vi "IHM_GetStringValue.vi"(4 "error in (no error)":errorcluster caption="entrée d'erreur (pas d'erreur)", 7 "Ref_IN":T1) -> (0 "Error out":errorcluster, 2 "StringValue":string, 3 "Ref_OUT":T1)   [LabVIEW 2013]
panel:
  out "ClassName":string
  out "Name":string
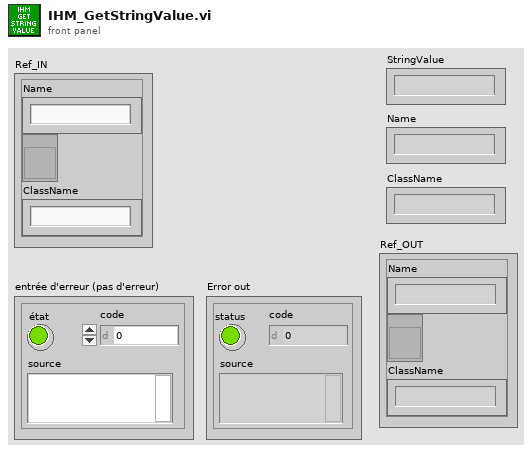
[diagram p1: front panel]
types:
  T1 = cluster{"Name":string, refnum<vi>, "ClassName":string}
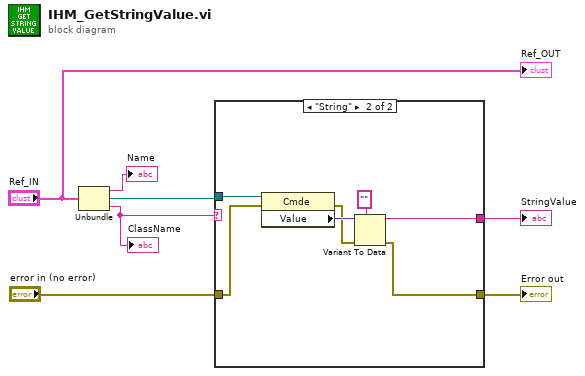
[diagram p0: block diagram]
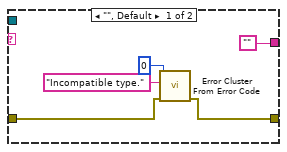
[diagram p2: hidden frame]
diagram:
  n1 = Unbundle("Ref_IN") -> ("Name"=→"Name":string, w6:refnum<vi>, "ClassName"=w7:string)
  "ClassName" <- w7
  n2 = case shown="\"String\"" w7 {
    tunnel: w6 -> [_ w18]
    tunnel: "error in (no error)" -> [w12 w17]
    tunnel: [w11 w15] -> w2
    tunnel: ["" w13] -> w1
    frame "", Default {
      n3 = call <vilib>:"Error Cluster From Error Code.vi"("error in (no error)"=w12, "error message (\"\")"="Incompatible type." ("error message (\"\")"), "error code (0)"=0) -> ("error out"=w11:errorcluster)  [unwired: 6 in]
    }
    frame "String" {
      n4 = property class="Cmde"(reference=w18, error in=w17) -> (error out=w16:errorcluster, "Value"=w19:variant)  [unwired: 1 out]
      n5 = Variant To Data(error in=w16, type="", Variant=w19) -> (data=w13:string, error out=w15:errorcluster)
    }
  }
  "Error out" <- w2
  "StringValue" <- w1
  "Ref_OUT" <- "Ref_IN"
